vi "Open Session Base.vi"(0 "eye scan in":refnum<class "niHighSpeedSerial Eye Scan v1 Host.lvclass">, 5 "instruction target":refnum<class "niInstr Instruction Target v1 Host.lvclass">, 7 "parent context":refnum<class "niInstr Instruction Framework Context v1 Host.lvclass">, 9 "instance(s)":u8[](array[numeric]), 11 "error in":errorcluster, 12 "select session":refnum<class "niHighSpeedSerial Eye Scan Single Point v1 Host.lvclass">) -> (4 "eye scan out":refnum<class "niHighSpeedSerial Eye Scan v1 Host.lvclass">, 15 "error out":errorcluster)   [LabVIEW 2016, in "niHighSpeedSerial Eye Scan v1 Host.lvclass"]
doc: "Creates the base class and initializes it to a good state.\n\n<B>Input Parameters</B>\n\n<B>eye scan in</B> Takes in a reference to your session from the previous VI.\n\n<B>instruction target</B> is the instruction target to use when communicating with the FPGA.\n\n<B>parent context</B> is the context of the parent instance. In most cases you can wire a default value.\n\n<B>instance(s)</B> The channel instances used.\n\n<B>error in</B> describes error conditions that occur before this node runs. This input provides standard 'error in' functionality.\n\n<B>Output Parameters</B>\n\n<B>eye scan out</B> passes a reference to your session to the next VI.\n\n<B>error out</B> contains error information. This output provides standard 'error out' functionality."
uses:
  <instrlib>/niHighSpeedSerial/Eye Scan/v1/Host/Eye Scan/niHighSpeedSerial Eye Scan v1 Host.lvclass
  <instrlib>/_niInstr/Instruction Framework/v1/Host/Instruction Target/niInstr Instruction Target v1 Host.lvclass
  <instrlib>/_niInstr/Instruction Framework/v1/Host/Instruction Framework Context/niInstr Instruction Framework Context v1 Host.lvclass
  <instrlib>/niHighSpeedSerial/Eye Scan/v1/Host/Impl/Single Point/niHighSpeedSerial Eye Scan Single Point v1 Host.lvclass
  <instrlib>/niHighSpeedSerial/Eye Scan/v1/Host/Eye Scan/Private/Private Data.ctl
  <instrlib>/niHighSpeedSerial/Eye Scan/v1/Host/Eye Scan/Private/Channel Data.ctl
  <instrlib>/niHighSpeedSerial/Eye Scan/v1/Host/Impl/Eye Scan Point Iterator/niHighSpeedSerial Eye Scan Point Iterator v1 Host.lvclass
  <instrlib>/niHighSpeedSerial/Eye Scan/v1/Host/Eye Scan/Private/Measure State.ctl
  <instrlib>/niHighSpeedSerial/Eye Scan/v1/Host/Common/Public/RX Output Divider.ctl
  <instrlib>/niHighSpeedSerial/Eye Scan/v1/Host/Common/Public/Equalization Mode.ctl
  <instrlib>/niHighSpeedSerial/Eye Scan/v1/Host/Common/Public/Data Width.ctl
  <instrlib>/niHighSpeedSerial/Eye Scan/v1/Host/Eye Scan/niHighSpeedSerial Eye Scan v1 Host.lvclass/niHighSpeedSerial Eye Scan v1 Host.ctl
  <vilib>/Utility/error.llb/Error Cluster From Error Code.vi
  <vilib>/ErrorRing/Error Ring.xnode
  <instrlib>/niHighSpeedSerial/Eye Scan/v1/Host/Common/niHighSpeedSerial Eye Scan Common v1 Host.lvlib
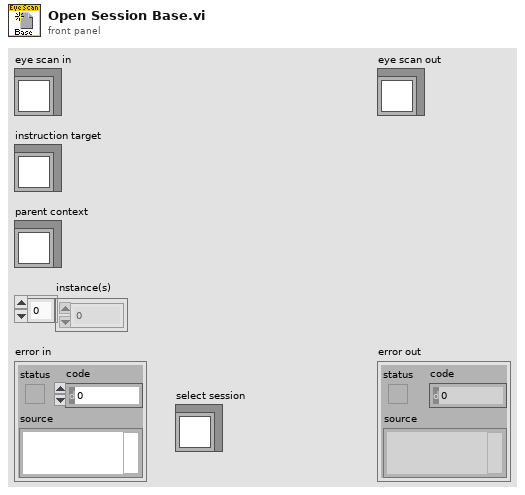
[diagram p1: front panel]
types:
  T1 = typedef "niHighSpeedSerial Eye Scan Common v1 Host.lvlib/RX Output Divider.ctl" = enum16{"1", "2", "4", "8", "16"}
  T2 = typedef "niHighSpeedSerial Eye Scan Common v1 Host.lvlib/Data Width.ctl" = enum16{"16 Bit", "20 Bit", "32 Bit", "40 Bit"}
  T3 = typedef "niHighSpeedSerial Eye Scan Common v1 Host.lvlib/Equalization Mode.ctl" = enum16{"DFE", "LPM"}
  T4 = typedef "niHighSpeedSerial Eye Scan v1 Host.lvclass/Measure State.ctl" = enum16{"Uninitialized", "Initialized", "Ready", "Measuring", "Finished", "Aborted"}
  T5 = typedef "niHighSpeedSerial Eye Scan v1 Host.lvclass/Private Data.ctl" = cluster{"instruction target":refnum<class "niInstr Instruction Target v1 Host.lvclass">, "channels":T6[], "measure state":T4, "rx output divider":T1, "equalization mode":T3, "rx internal data width":T2, "BER floor":dbl, "number of points completed":i32, "rx output divider configured?":bool, "equalization mode configured?":bool, "rx data width configured?":bool}
  T6 = typedef "niHighSpeedSerial Eye Scan v1 Host.lvclass/Channel Data.ctl" = cluster{"instance":u8, "channel":refnum<class "niHighSpeedSerial Eye Scan Single Point v1 Host.lvclass">, "point iterator":refnum<class "niHighSpeedSerial Eye Scan Point Iterator v1 Host.lvclass">}
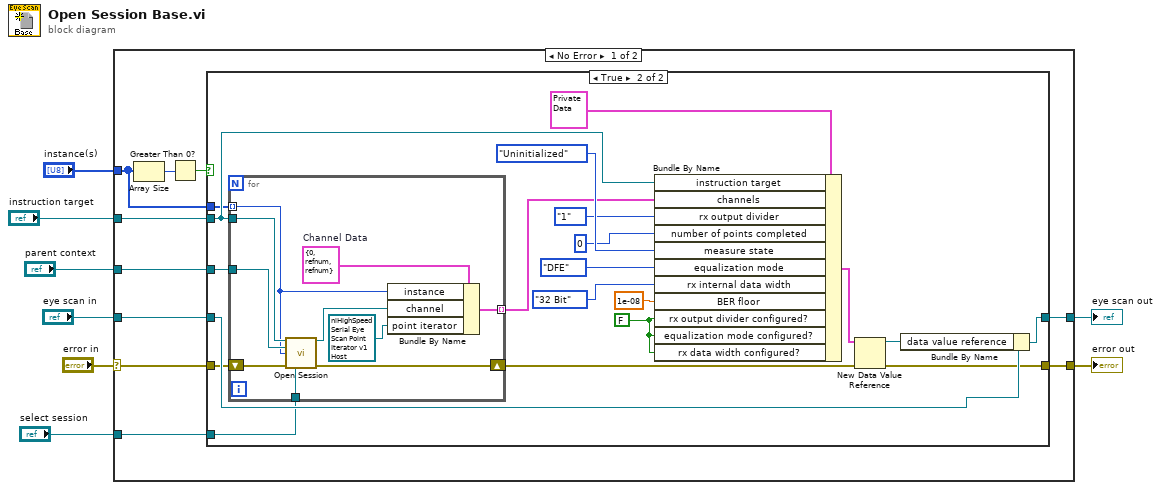
[diagram p0: block diagram]
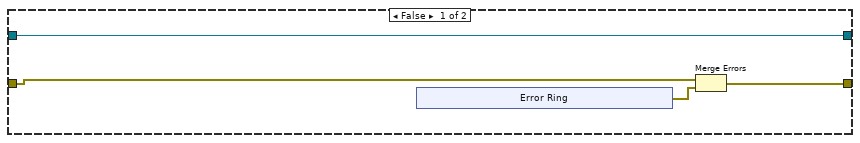
[diagram p2: hidden frame]
diagram:
  n1 = case shown="No Error" "error in" {
    selector: "error in" -> [w15 w58]
    tunnel: [w16 w58] -> w7
    tunnel: "eye scan in" -> [w18 w57]
    tunnel: [w17 w57] -> w5
    tunnel: "instance(s)" -> [w12 _]
    tunnel: "parent context" -> [w14 _]
    tunnel: "instruction target" -> [w13 _]
    tunnel: "select session" -> [w9 _]
    frame No Error {
      n2 = Array Size(array=w12) -> (size(s)=w11:i32)
      n3 = Greater Than 0?(x=w11) -> (x > 0?=w10:bool)
      n4 = case shown="True" w10 {
        tunnel: w18 -> [w22 w46]
        tunnel: [w22 w45] -> w17
        tunnel: [w20 w41] -> w16
        tunnel: w15 -> [w21 w40]
        tunnel: w14 -> [_ w38]
        tunnel: w13 -> [_ w37]
        tunnel: w12 -> [_ w30]
        tunnel: w9 -> [_ w27]
        frame False {
          n5 = xnode "Error Ring"() -> ("error out"=w19:errorcluster)
          n6 = Merge Errors(w21, w19) -> (w20:errorcluster)
        }
        frame True {
          w28 = FALSE ("rx output divider configured?")
          n7 = for {
            tunnel: w37 -> [w54]
            tunnel: w38 -> [w53]
            shift-right: [w55] -> w39
            shift-left: w40 -> [w56]
            tunnel: w30 -> [w48] mode=indexing
            tunnel: [w51] -> w34 mode=indexing
            tunnel: w27 -> [w47]
            w50 = T6 {"instance"=0, "channel"=refnum, "point iterator"=refnum}  # Channel Data
            n8 = call-dynamic "Open Session.vi"("instruction target"=w54, "parent context"=w53, "channel instance"=w48, "error in"=w56, "select session"=w47) -> ("eye scan single point out"=w52:refnum<class "niHighSpeedSerial Eye Scan Single Point v1 Host.lvclass">, "error out"=w55:errorcluster)  [unwired: 9 in]
            n9 = Bundle By Name(cluster=w50, "instance"=w48, "channel"=w52, "point iterator"=refnum<class "niHighSpeedSerial Eye Scan Point Iterator v1 Host.lvclass"> refnum ("Point Iterator")) -> (w51:T6)
          }
          n10 = Bundle By Name(cluster=T5 {"instruction target"=refnum, "channels"=[], "measure state"=enum."Uninitialized", "rx output divider"=enum."1", "equalization mode"=enum."DFE", "rx internal data width"=enum."32 Bit", "BER floor"=0.0, "number of points completed"=0, "rx output divider configured?"=FALSE, "equalization mode configured?"=FALSE, "rx data width configured?"=FALSE} ("Cluster"), "instruction target"=w37, "channels"=w34, "rx output divider"=RX_Output_Divider."1", "number of points completed"=0 ("Number of Points Completed"), "measure state"=Measure_State."Uninitialized" ("Measure State"), "equalization mode"=Equalization_Mode."DFE" ("Equalization Mode"), "rx internal data width"=Data_Width."32 Bit" ("data width"), "BER floor"=1e-08 ("BER Floor"), "rx output divider configured?"=w28, "equalization mode configured?"=w28, "rx data width configured?"=w28) -> (w43:T5)
          n11 = New Data Value Reference(data value=w43, error in=w39) -> (data value reference=w42:refnum<data-value>, error out=w41:errorcluster)
          n12 = Bundle By Name(cluster=w46, "data value reference"=w42) -> (w45:refnum<class "niHighSpeedSerial Eye Scan v1 Host.lvclass">)
        }
      }
    }
    frame Error {
    }
  }
  "error out" <- w7
  "eye scan out" <- w5
